vi "Get Accessibility.vi"(8 "error in (no error)":errorcluster, 11 "SMO":refnum<class "SMO.lvclass">) -> (0 "error out":errorcluster, 2 "Accessibility":T1, 3 "SMO out":refnum<class "SMO.lvclass">)   [LabVIEW 2019, in "SMO.lvclass"]
doc: "JKI State Machine Objects (SMO) 1.3.0.56\nJKI - JKI\nCopyright (c) 2017, JKI"
uses:
  SMO.lvclass
  Typedefs/Accessibility--Cluster.ctl
  Typedefs/Reserve State--Enum.ctl
  SMO.lvclass/SMO.ctl
panel:
  # "For instructions on how to use the JKI State Machine Objects, examples and video tutorials, visit:\nhttp://jki.net/state-machine-objects/\n\nJKI State Machine Objects™\nhttp://jki.net/state-machine-objects/\nCopyright (C) 2005-2015, JKI <info@jki.net>\nALL RIGHTS RESERVED"
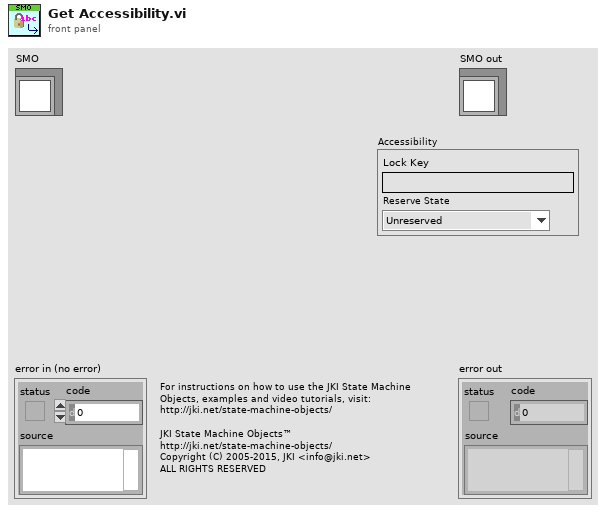
[diagram p1: front panel]
types:
  T1 = typedef "SMO.lvclass/Accessibility--Cluster.ctl" = cluster{"Lock Key":string, "Reserve State":T2}
  T2 = typedef "SMO.lvclass/Reserve State--Enum.ctl" = enum16{"Unreserved", "Reserved", "Self-locked"}
  T3 = typedef "SMO.lvclass/PrivateData--Ref.ctl" = refnum<data-value>
  T4 = typedef "SMO.lvclass/PrivateData--Cluster.ctl" = cluster{"Parent Call":T5, "Registered Processes":T6[], "Sync Notifier":refnum<notifier>, "Process Error Notifier":refnum<notifier>, "Protected Events":T7, "Public Events":T8, "SMO State":T9, "[Dependencies]":T10[], "[Attributes]":refnum<class "Attribute.lvclass">[], "Launcher Close":refnum<notifier>, "Caller Watchdog":refnum<queue>, "Accessibility":T1, "NbStaticDependencies":u32}
  T5 = typedef "SMO.lvclass/Parent Call--Enum.ctl" = enum16{"Allows parent to run", "Does not request parent to run"}
  T6 = typedef "SMO.lvclass/RegisteredProcessData--Cluster.ctl" = cluster{"Name":string, "Static VI Ref":refnum<vi>, "Running":bool, "NotifierRef":u32}
  T7 = typedef "SMO.lvclass/Protected Events.ctl" = cluster{"StopProcesses":refnum<user-event>, "AbortProcesses":refnum<user-event>, "Config Changed":refnum<user-event>, "Dependency":refnum<user-event>}
  T8 = typedef "SMO.lvclass/Public Events.ctl" = cluster{"Error":refnum<user-event>, "State":refnum<user-event>, "Reserve State":refnum<user-event>}
  T9 = typedef "SMO.lvclass/SMOState --Enum.ctl" = enum16{"unknown", "Created", "Started", "Stopped"}
  T10 = typedef "SMO.lvclass/SMO Dependency--Cluster.ctl" = cluster{"Dependency":refnum<class "SMO.lvclass">, "Level":string}
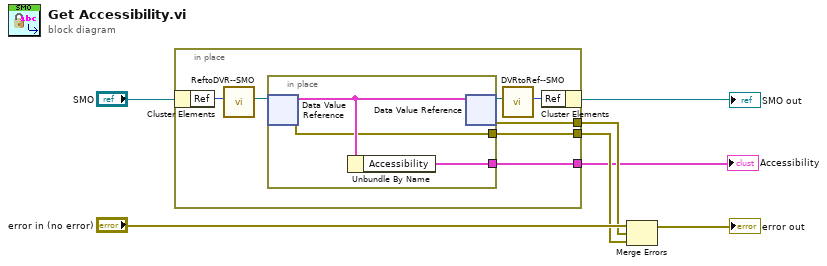
[diagram p0: block diagram]
diagram:
  n1 = in-place {
    in-place-border: [w14] -> w1
    in-place-border: [w13] -> w2
    in-place-border: [w12] -> w3
    n2 = in-place-cluster #1("SMO") -> ("Ref"=w11:u32)
    n3 = call "ReftoDVR--SMO.vi"("Ref"=w11) -> ("Ref"=w10:T3)  [unwired: 10 in]
    n4 = in-place {
      in-place-border: [w17] -> w14
      in-place-border: [w15] -> w12
      n5 = in-place-dvr #2(w10) -> (w16:T4, w15:errorcluster)
      n6 = Unbundle By Name(w16) -> ("Accessibility"=w17:T1)
      n7 = in-place-dvr #2(w16) -> (w9:T3, w13:errorcluster)
    }
    n8 = call "DVRtoRef--SMO.vi"("Ref"=w9) -> ("Ref"=w8:u32)  [unwired: 10 in]
    n9 = in-place-cluster #1("Ref"=w8) -> (→"SMO out":refnum<class "SMO.lvclass">)
  }
  "Accessibility" <- w1
  n10 = Merge Errors("error in (no error)", w2, w3) -> (→"error out":errorcluster)
